vi "Get_Test_File_Path.vi"(11 "path":path) -> (2 "选中文件:":string)   [LabVIEW 2018]
uses:
  Global.vi
panel:
  in  "stop":bool caption="停止"
  in  "OK":bool caption="元素入队列"
  out "数组":string[](array[string])
  in  "文件列表":i32(listbox)
  out "文件名":string[](array[string])
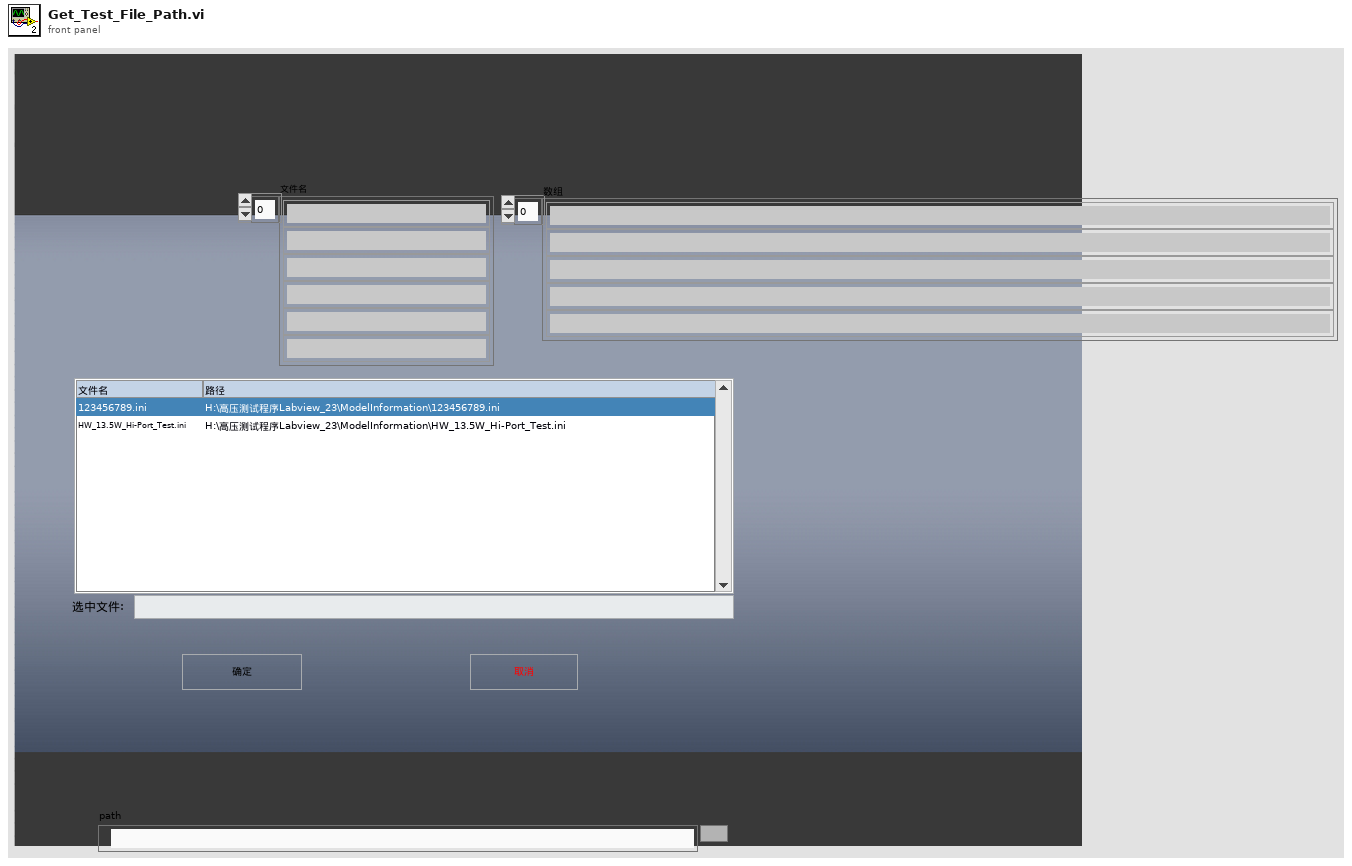
[diagram p1: front panel]
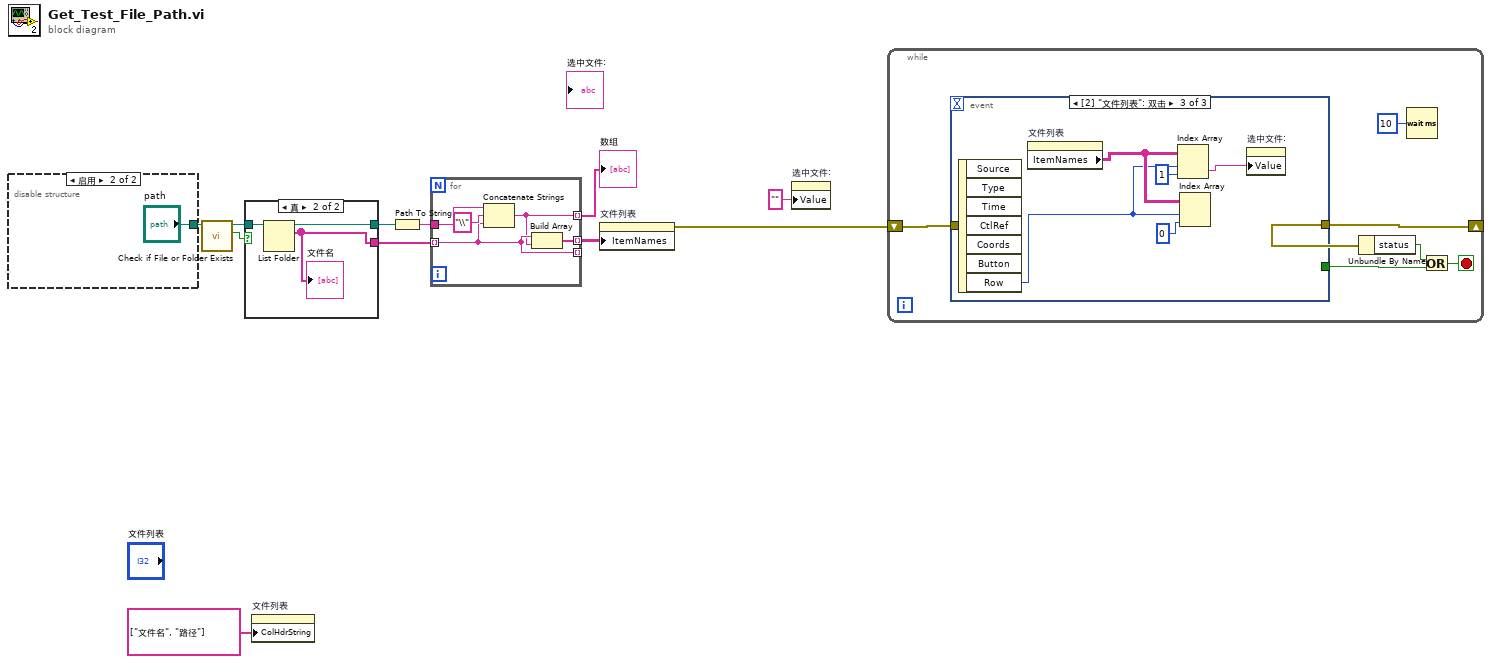
[diagram p0: block diagram]
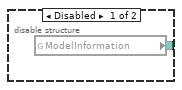
[diagram p2: hidden frame]
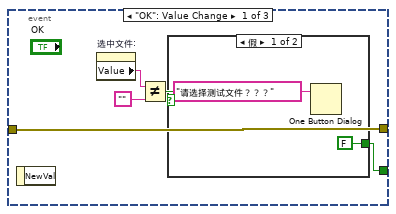
[diagram p3: hidden frame]
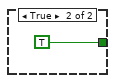
[diagram p4: hidden frame]
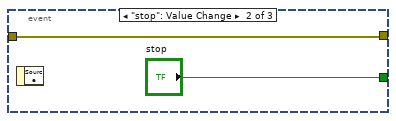
[diagram p5: hidden frame]
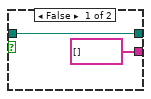
[diagram p6: hidden frame]
diagram:
  n1 = disable-structure shown="启用" {
    disable-tunnel: [w12 "path"] -> w11
    frame Disabled {
      n2 = global read "Global.vi" "ModelInformation"() -> (w12:path)
    }
    frame Enabled {
    }
  }
  n3 = call <vilib>:"Check if File or Folder Exists.vi"("path"=w11) -> ("file or folder exists?"=w10:bool, "dup path"=w9:path)  [unwired: 8 in, 1 out]
  n4 = case shown="真" w10 {
    tunnel: w9 -> [w14 w18]
    tunnel: [string[] [] ("filenames") w17] -> w6
    tunnel: [w14 w16] -> w7
    frame False {
    }
    frame True {
      n5 = List Folder(path=w18) -> (path out=w16:path, filenames=w17:string[])  [unwired: 3 in, 2 out]
      "文件名" <- w17
    }
  }
  n6 = property on="文件列表" class="MCListbox (严格)"("ColHdrString"=string[] ["文件名", "路径"] ("列首字符串[]")) -> ()  [unwired: 2 in, 2 out]
  n7 = Path To String(path=w7) -> (string=w5:string)
  n8 = for {
    tunnel: w6 -> [w21] mode=indexing
    tunnel: w5 -> [w23]
    tunnel: [w20] -> w4 mode=indexing
    tunnel: [w21] -> _ mode=indexing
    tunnel: [w19] -> w3 mode=indexing
    n9 = Concatenate Strings(w23, "\\" ("字符串"), w21) -> (w20:string)
    n10 = Build Array(w21, w20) -> (w19:string[])
  }
  "数组" <- w4
  n11 = property on="文件列表" class="MCListbox (严格)"("ItemNames"=w3) -> (error out=w2:errorcluster)  [unwired: 2 in, 1 out]
  n12 = property on="选中文件:" class="Str"("Value"="" ("选中文件:")) -> ()  [unwired: 2 in, 2 out]
  n13 = while {
    shift-right: [w26] -> _
    shift-left: w2 -> [w29]
    stop <- w27 stop-if-true
    n14 = event shown="[2] \"文件列表\": 双击" {
      selector: _ -> [_ _ _]
      dyn-events: _ -> [_ _ _]
      timeout: _ -> [_ _ _]
      tunnel: w29 -> [w34 w38 _]
      tunnel: [w34 w38 _] -> w26
      tunnel: [w30 "stop" _] -> w28
      event "OK": Value Change {
        n15 = event-data() -> ()  [unwired: 1 in, 1 out]
        n16 = property on="选中文件:" class="Str"() -> ("Value"=w33:string)  [unwired: 2 in, 2 out]
        n17 = Not Equal?(x=w33, y="") -> (x != y?=w31:bool)
        n18 = case shown="假" w31 {
          tunnel: [FALSE TRUE] -> w30
          frame False {
            n19 = One Button Dialog(message="请选择测试文件？？？" ("消息")) -> ()  [unwired: 1 in, 1 out]
          }
          frame True {
          }
        }
      }
      event "stop": Value Change {
        n20 = event-data() -> ()  [unwired: 1 in, 1 out]
      }
      event "文件列表": Double Click {
        n21 = event-data() -> ("Row"=w41:i32)  [unwired: 1 in, 6 out]
        n22 = property on="文件列表" class="MCListbox (严格)"() -> ("ItemNames"=w42:string[][])  [unwired: 2 in, 2 out]
        n23 = Index Array(array=w42, index (row)=w41, index (col)=1 ("禁用的索引 (列)")) -> (element=w40:string)
        n24 = Index Array(array=w42, index (row)=w41, index (col)=0 ("禁用的索引 (列)")) -> ()  [unwired: 1 out]
        n25 = property on="选中文件:" class="Str"("Value"=w40) -> ()  [unwired: 2 in, 2 out]
      }
    }
    n26 = Unbundle By Name(w26) -> ("status"=w25:bool)
    n27 = Wait (ms)(milliseconds to wait=u32 10 ("等待时间（毫秒）")) -> ()  [unwired: 1 out]
    n28 = Or(x=w25, y=w28) -> (x .or. y?=w27:bool)
  }
